vi "FlatToRichni_bus_monitor_api_ResetStreamingFilterReply.vi"(5 "OutputClusterType":T1, 11 "InputCluster":T6) -> (3 "OutputCluster":T1)   [LabVIEW 2025, in "bus_monitor_server.lvlib"]
uses:
  bus_monitor_server.lvlib
  ni_bus_monitor_api_ResetStreamingFilterReply_Flat.ctl
  ni_bus_monitor_api_FilterInfo_Flat.ctl
  ni_bus_monitor_api_DirectionFilter.ctl
  ni_bus_monitor_api_FrameFilter.ctl
  ni_bus_monitor_api_ErrorInfo_Flat.ctl
  ni_bus_monitor_api_ResetStreamingFilterReply.ctl
  ni_bus_monitor_api_FilterInfo.ctl
  ni_bus_monitor_api_ErrorInfo.ctl
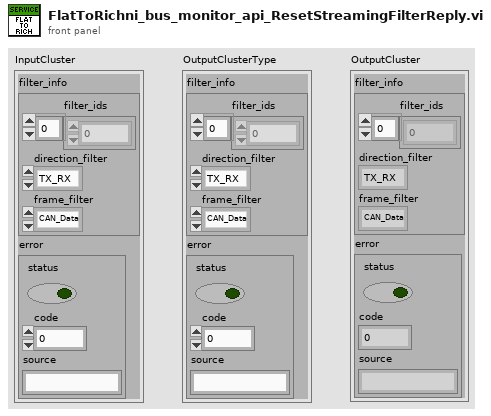
[diagram p1: front panel]
types:
  T1 = typedef "bus_monitor_server.lvlib/ni_bus_monitor_api_ResetStreamingFilterReply.ctl" = cluster{"filter_info":T2, "error":T5}
  T2 = typedef "bus_monitor_server.lvlib/ni_bus_monitor_api_FilterInfo.ctl" = cluster{"filter_ids":u32[], "direction_filter":T3, "frame_filter":T4}
  T3 = typedef "bus_monitor_server.lvlib/ni_bus_monitor_api_DirectionFilter.ctl" = enum32{"TX_RX", "RX", "TX"}
  T4 = typedef "bus_monitor_server.lvlib/ni_bus_monitor_api_FrameFilter.ctl" = enum32{"CAN_Data", "CAN_Remote", "CAN_Bus_Error", "CAN_2_Data", "CAN_FD_Data", "CAN_FD_BRS_Data", "J1939_Data", "Delay", "Log_Trigger", "Start_Trigger", "All"}
  T5 = typedef "bus_monitor_server.lvlib/ni_bus_monitor_api_ErrorInfo.ctl" = errorcluster
  T6 = typedef "bus_monitor_server.lvlib/ni_bus_monitor_api_ResetStreamingFilterReply_Flat.ctl" = cluster{"filter_info":T7, "error":T8}
  T7 = typedef "bus_monitor_server.lvlib/ni_bus_monitor_api_FilterInfo_Flat.ctl" = cluster{"filter_ids":u32[], "direction_filter":T3, "frame_filter":T4}
  T8 = typedef "bus_monitor_server.lvlib/ni_bus_monitor_api_ErrorInfo_Flat.ctl" = errorcluster
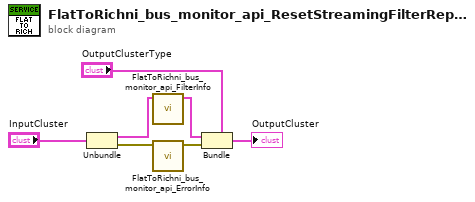
[diagram p0: block diagram]
diagram:
  n1 = Unbundle "Unbundle"("InputCluster") -> ("filter_info"=w4:T7, "error"=w2:T8)
  n2 = call "FlatToRichni_bus_monitor_api_FilterInfo.vi"("InputCluster"=w4) -> ("OutputCluster"=w3:T2)  [unwired: 10 in]
  n3 = call "FlatToRichni_bus_monitor_api_ErrorInfo.vi"("InputCluster"=w2) -> ("OutputCluster"=w1:T5)  [unwired: 10 in]
  n4 = Bundle "Bundle"(cluster="OutputClusterType", "filter_info"=w3, "error"=w1) -> (→"OutputCluster":T1)
